vi "数据全参数一起发送整点触发.vi"(6 "数据发送通道":enum16{"TCP", "VISA"}(ring), 8 "PW":string, 9 "MN":string) -> ()   [LabVIEW 2016, in "数据传输系统.lvlib"]
panel:
  out "table":string="提取小时数据"
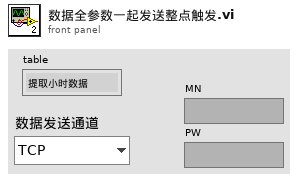
[diagram p1: front panel]
types:
  T1 = typedef "LVDateTimeRec.ctl" = cluster{"秒数的小数部分":dbl, "秒":i32, "分":i32, "时":i32, "日":i32, "月":i32, "年":i32, "天数（周）":i32, "天数（年）":i32, "DST":i32}
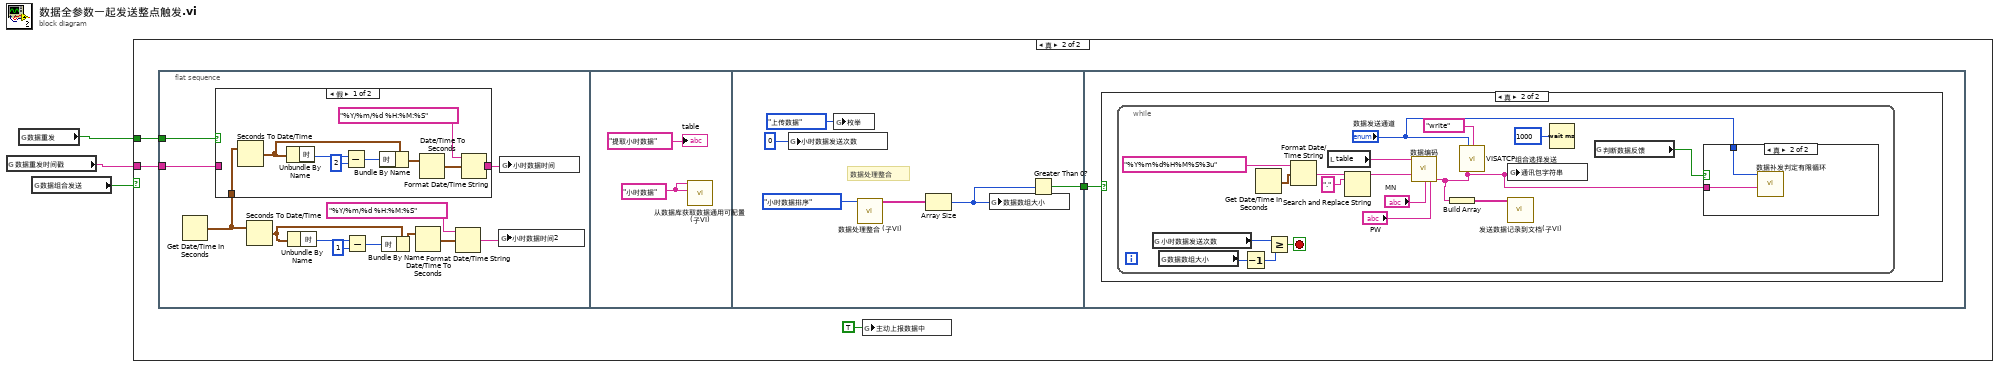
[diagram p0: block diagram]
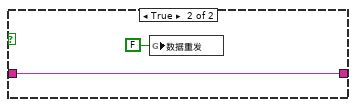
[diagram p3: hidden frame]
diagram:
  n1 = global read "断电保存全局.vi" "数据重发时间戳"() -> (w1:string)
  n2 = global read "断电保存全局.vi" "数据重发"() -> (w2:bool)
  n3 = global read "断电保存全局.vi" "数据组合发送"() -> (w3:bool)
  n4 = case shown="真" w3 {
    tunnel: w2 -> [_ w6]
    tunnel: w1 -> [_ w5]
    frame False {
    }
    frame True {
      n5 = flat-sequence {
        tunnel: w6 -> [w14]
        tunnel: w5 -> [w13]
        tunnel: [w34] -> w7
        tunnel: w7 -> [w39]
        frame #0 {
          n6 = Get Date/Time In Seconds() -> (seconds since 1Jan1904=w19:timestamp)
          n7 = case shown="假" w14 {
            tunnel: w19 -> [w28 _]
            tunnel: [w20 w30] -> w16
            tunnel: w13 -> [_ w30]
            frame False {
              n8 = Seconds To Date/Time(time stamp (now)=w28) -> (date time rec=w23:T1)  [unwired: 1 in]
              n9 = Unbundle By Name(w23) -> ("时"=w21:i32)
              n10 = Subtract(x=w21, y=2) -> (x-y=w24:i32)
              n11 = Bundle By Name(cluster=w23, "时"=w24) -> (w25:T1)
              n12 = Date/Time To Seconds(2:w25) -> (0:w26:timestamp)  [unwired: 1 in]
              n13 = Format Date/Time String(time format string (%c)="%Y/%m/%d %H:%M:%S" ("时间格式字符串(%c)"), seconds (now)=w26) -> (date/time string=w20:string)  [unwired: 1 in]
            }
            frame True {
              n14 = global write "断电保存全局.vi" "数据重发"(FALSE ("数据重发")) -> ()
            }
          }
          n15 = Seconds To Date/Time(time stamp (now)=w19) -> (date time rec=w9:T1)  [unwired: 1 in]
          n16 = Unbundle By Name(w9) -> ("时"=w12:i32)
          n17 = Subtract(x=w12, y=1) -> (x-y=w10:i32)
          n18 = Bundle By Name(cluster=w9, "时"=w10) -> (w8:T1)
          n19 = Date/Time To Seconds(2:w8) -> (0:w18:timestamp)  [unwired: 1 in]
          n20 = Format Date/Time String(time format string (%c)="%Y/%m/%d %H:%M:%S" ("时间格式字符串(%c)"), seconds (now)=w18) -> (date/time string=w15:string)  [unwired: 1 in]
          n21 = global write "全局 时间2.vi" "小时数据时间2"(w15) -> ()
          n22 = global write "全局 水样时间.vi" "小时数据时间"(w16) -> ()
        }
        frame #1 {
          w32 = "小时数据" ("名称（未命名）")
          n23 = call "从数据库获取数据通用可配置(子VI).vi"("table输入"=w32, "列队名（唯一）"=w32) -> ()  [unwired: 8 in, 2 out]
          "table" <- "提取小时数据" ("新元素/子数组")
        }
        frame #2 {
          # "数据处理整合"
          n24 = global write "全局 小时数据发送次数.vi" "小时数据发送次数"(0 ("数值")) -> ()
          n25 = global write "全局1.vi" "枚举"(enum16{"返回请求应答", "上传数据", "返回执行结果"}."上传数据" ("枚举")) -> ()
          n26 = call "数据处理整合 (子VI).vi"("枚举"=enum16{"实时数据排序", "小时数据排序"}."小时数据排序") -> ("已排序的数组"=w38:string[])  [unwired: 10 in]
          n27 = Array Size(array=w38) -> (size(s)=w35:i32)
          n28 = global write "全局 数据数组大小.vi" "数据数组大小"(w35) -> ()
          n29 = Greater Than 0?(x=w35) -> (x > 0?=w34:bool)
        }
        frame #3 {
          n30 = case shown="真" w39 {
            frame False {
            }
            frame True {
              n31 = while {
                stop <- w54 stop-if-true
                n32 = global read "全局 小时数据发送次数.vi" "小时数据发送次数"() -> (w57:i32)
                n33 = global read "全局 数据数组大小.vi" "数据数组大小"() -> (w48:i32)
                n34 = Decrement(x=w48) -> (x-1=w49:i32)
                n35 = Get Date/Time In Seconds() -> (seconds since 1Jan1904=w45:timestamp)
                n36 = Greater Or Equal?(x=w57, y=w49) -> (x >= y?=w54:bool)
                n37 = Format Date/Time String(time format string (%c)="%Y%m%d%H%M%S%3u" ("时间格式字符串(%c)"), seconds (now)=w45) -> (date/time string=w46:string)  [unwired: 1 in]
                n38 = local read "table"() -> (w53:string)
                n39 = Search and Replace String(input string=w46, search string="." ("搜索字符串")) -> (result string=w43:string)  [unwired: 6 in, 3 out]
                n40 = call "数据编码.vi"("table输入"=w53, "QN"=w43, "MN"="MN", "PW"="PW") -> ("通讯包字符串"=w40:string)  [unwired: 10 in, 1 out]
                n41 = Build Array(w40) -> (w56:string[])
                n42 = call "VISATCP组合选择发送.vi"("数据发送通道"="数据发送通道", "命令"="write", "写入缓冲区"=w40) -> ()  [unwired: 9 in, 4 out]
                n43 = global write "全局1.vi" "通讯包字符串"(w40) -> ()
                n44 = call "发送数据记录到文档(子VI).vi"("数组"=w56) -> ()  [unwired: 9 in, 1 out]
                n45 = Wait (ms)(milliseconds to wait=u32 1000 ("等待时间（毫秒）")) -> ()  [unwired: 1 out]
                n46 = global read "断电保存全局.vi" "判断数据反馈"() -> (w42:bool)
                n47 = case shown="真" w42 {
                  tunnel: "数据发送通道" -> [_ w59]
                  tunnel: w40 -> [_ w58]
                  frame False {
                  }
                  frame True {
                    n48 = call "数据补发判定有限循环.vi"("数据输入"=w58, "数据发送通道"=w59) -> ()  [unwired: 9 in, 1 out]
                  }
                }
              }
            }
          }
        }
      }
      n49 = global write "全局 数据发送重叠.vi" "主动上报数据中"(TRUE ("主动上报数据中")) -> ()
    }
  }
